vi "PORT IO Write__ogtk.vi"   [LabVIEW 2020]
doc: "This function writes data to the specified IO port. If you set fast to True, and are running under Windows NT/2000/XP/2003 you must have enabled the according IO port with a call to \"PORT IO Enable Range.vi\" to avoid a General Protection Fault error."
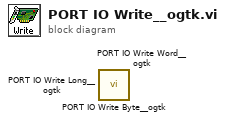
[diagram p0: block diagram]
diagram:
  n1 = call <userlib>:"PORT IO Write Byte__ogtk.vi"() -> ()  [unwired: 7 in, 1 out]
  n2 = call <userlib>:"PORT IO Write Word__ogtk.vi"() -> ()  [unwired: 7 in, 1 out]
  n3 = call <userlib>:"PORT IO Write Long__ogtk.vi"() -> ()  [unwired: 7 in, 1 out]
